vi "Drop Parameters.vi"(6 "Main UI Message Queue":refnum<queue>, 7 "Mouse Position":cluster{"X":i32, "Y":i32}, 8 "error in (no error)":errorcluster, 9 "Parent Window Title":string, 10 "Module Type":T1=enum."Feed", 11 "State in":T2 {"Main Config"."PR Module Configs"."Settings"."PID 2 Parameters"."output range"."output low" format="%.2f"; "Main Config"."PR Module Configs"."Settings"."PID 2 Parameters"."output range"."output high" min=0.0 max=100.0 format="%.2f"; "Main Config"."PR Module Configs"."Settings"."PID 2 Parameters"."PID gains"."derivative time (Td, min)" format="%.3f"; "Main Config"."PR Module Configs"."Settings"."PID 2 Parameters"."PID gains"."integral time (Ti, min)" format="%.3f"; "Main Config"."PR Module Configs"."Settings"."PID 2 Parameters"."PID gains"."proportional gain (Kc)" format="%.3f"; "Main Config"."Steps"."Control" items=["Pump %", "Setpoint"]; "Main Config"."TCU Module Configs"."Settings"."Huber Unistat 410 Settings"."Address" min=0 max=99 format="%02.0f"; "Main Config"."TCU Module Configs"."Settings"."Julabo FP-50 Settings"."Pump Power" min=0 max=8 step=1; "Main Config"."TCU Module Configs"."Settings"."Lauda Settings"."Pump Power" min=0 max=8 step=1; "Main Config"."Flow Module Configs"."Settings"."Bronkhorst M14 Settings"."Smoothing Steps" min=1 step=1; "Main Config"."Flow Module Configs"."Settings"."Bronkhorst M13 Settings"."Smoothing Steps" min=1 step=1; "Main Config"."Pump Module Configs"."Settings"."Ismatech 3 Channel Settings"."Channel Number" min=0 max=3; "Main Config"."Pump Module Configs"."Settings"."Ismatech 3 Channel Settings"."Pump Number" min=1; "Main Config"."Pump Module Configs"."Settings"."ASIA Pump C"."channel" min=0 max=1 step=1; "Main Config"."Pump Module Configs"."Settings"."Masterflex"."Pump Number" min=1.0 max=20.0 step=1.0; "Main Config"."Pump Module Configs"."Settings"."Ismatech"."Pump Number" min=1.0 max=20.0 step=1.0; "Main Config"."Feed Module Configs"."Settings"."Bronkhorst M14 Settings"."Smoothing Steps" min=1 step=1; "Main Config"."Feed Module Configs"."Settings"."Ismatech 3 Channel Settings"."Channel Number" min=0 max=3; "Main Config"."Feed Module Configs"."Settings"."Ismatech 3 Channel Settings"."Pump Number" min=1; "Main Config"."Feed Module Configs"."Settings"."PID range"."PID Low" min=0.0 max=100.0 format="%.2f"; "Main Config"."Feed Module Configs"."Settings"."PID range"."PID High" format="%.2f"; "Main Config"."Feed Module Configs"."Settings"."PID 2 Parameters"."PID gains"."derivative time (Td, min)" format="%.3f"; "Main Config"."Feed Module Configs"."Settings"."PID 2 Parameters"."PID gains"."integral time (Ti, min)" format="%.3f"; "Main Config"."Feed Module Configs"."Settings"."PID 2 Parameters"."PID gains"."proportional gain (Kc)" format="%.3f"; "Main Config"."Feed Module Configs"."Settings"."Bronkhorst M13 Flow Meter"."Smoothing Steps" min=1 step=1; "Main Config"."Feed Module Configs"."Settings"."ASIA Pump C"."channel" min=0 max=1 step=1; "Main Config"."Feed Module Configs"."Settings"."Ismatech"."Pump Number" min=1.0 max=20.0 step=1.0; "Main Config"."Feed Module Configs"."Settings"."Masterflex"."Pump Number" min=1.0 max=20.0 step=1.0}) -> (0 "error out":errorcluster, 2 "Drop Parameters":T79, 3 "State out":T2 {"Main Config"."PR Module Configs"."Settings"."PID 2 Parameters"."output range"."output low" format="%.2f"; "Main Config"."PR Module Configs"."Settings"."PID 2 Parameters"."output range"."output high" min=0.0 max=100.0 format="%.2f"; "Main Config"."PR Module Configs"."Settings"."PID 2 Parameters"."PID gains"."derivative time (Td, min)" format="%.3f"; "Main Config"."PR Module Configs"."Settings"."PID 2 Parameters"."PID gains"."integral time (Ti, min)" format="%.3f"; "Main Config"."PR Module Configs"."Settings"."PID 2 Parameters"."PID gains"."proportional gain (Kc)" format="%.3f"; "Main Config"."Steps"."Control" items=["Pump %", "Setpoint"]; "Main Config"."TCU Module Configs"."Settings"."Huber Unistat 410 Settings"."Address" min=0 max=99 format="%02.0f"; "Main Config"."TCU Module Configs"."Settings"."Julabo FP-50 Settings"."Pump Power" min=0 max=8 step=1; "Main Config"."TCU Module Configs"."Settings"."Lauda Settings"."Pump Power" min=0 max=8 step=1; "Main Config"."Flow Module Configs"."Settings"."Bronkhorst M14 Settings"."Smoothing Steps" min=1 step=1; "Main Config"."Flow Module Configs"."Settings"."Bronkhorst M13 Settings"."Smoothing Steps" min=1 step=1; "Main Config"."Pump Module Configs"."Settings"."Ismatech 3 Channel Settings"."Channel Number" min=0 max=3; "Main Config"."Pump Module Configs"."Settings"."Ismatech 3 Channel Settings"."Pump Number" min=1; "Main Config"."Pump Module Configs"."Settings"."ASIA Pump C"."channel" min=0 max=1 step=1; "Main Config"."Pump Module Configs"."Settings"."Masterflex"."Pump Number" min=1.0 max=20.0 step=1.0; "Main Config"."Pump Module Configs"."Settings"."Ismatech"."Pump Number" min=1.0 max=20.0 step=1.0; "Main Config"."Feed Module Configs"."Settings"."Bronkhorst M14 Settings"."Smoothing Steps" min=1 step=1; "Main Config"."Feed Module Configs"."Settings"."Ismatech 3 Channel Settings"."Channel Number" min=0 max=3; "Main Config"."Feed Module Configs"."Settings"."Ismatech 3 Channel Settings"."Pump Number" min=1; "Main Config"."Feed Module Configs"."Settings"."PID range"."PID Low" min=0.0 max=100.0 format="%.2f"; "Main Config"."Feed Module Configs"."Settings"."PID range"."PID High" format="%.2f"; "Main Config"."Feed Module Configs"."Settings"."PID 2 Parameters"."PID gains"."derivative time (Td, min)" format="%.3f"; "Main Config"."Feed Module Configs"."Settings"."PID 2 Parameters"."PID gains"."integral time (Ti, min)" format="%.3f"; "Main Config"."Feed Module Configs"."Settings"."PID 2 Parameters"."PID gains"."proportional gain (Kc)" format="%.3f"; "Main Config"."Feed Module Configs"."Settings"."Bronkhorst M13 Flow Meter"."Smoothing Steps" min=1 step=1; "Main Config"."Feed Module Configs"."Settings"."ASIA Pump C"."channel" min=0 max=1 step=1; "Main Config"."Feed Module Configs"."Settings"."Ismatech"."Pump Number" min=1.0 max=20.0 step=1.0; "Main Config"."Feed Module Configs"."Settings"."Masterflex"."Pump Number" min=1.0 max=20.0 step=1.0})   [LabVIEW 2018, in "Drag and Drop.lvlib"]
uses:
  Drag and Drop.lvlib
  Drop Parameters Cluster.ctl
  support/Message Queue/Message Cluster.ctl
  <vilib>/Utility/miscctls.llb/LVPoint32TypeDef.ctl
  State Cluster.ctl
  Thumbnail Cluster.ctl
  Object Cluster.ctl
  <vilib>/Utility/miscctls.llb/LVRectTypeDef.ctl
  Object Type Enum.ctl
  <vilib>/Utility/miscctls.llb/LVPositionTypeDef.ctl
  Config Module/Controls/Main Config Cluster.ctl
  OPC/OPC Module Config.ctl
  Scale Module Folder/Measure Instrument/State Enum.ctl
  OPC/OPC Settings.ctl
  OPC/Variable Data Cluster.ctl
  <vilib>/OPCUA/controls/NodeId.ctl
  <vilib>/OPCUA/controls/OPC UA StatusCode.ctl
  <vilib>/OPCUA/controls/Subscription ID.ctl
  <vilib>/OPCUA/controls/OPC UA Client Refnum.ctl
  <vilib>/OPCUA/controls/Subscription Data Change.ctl
  <vilib>/OPCUA/controls/Data Type.ctl
  OPC/OPC Tag Data.ctl
  Feed Module/Controls/Feed Module Config Cluster.ctl
  Feed Module/Controls/Feed Module Settings Cluster.ctl
  Ismatec ISM 831C/Controls/Ismatech ISM831C Settings Cluster.ctl
  Masterflex 7550-30/Controls/Settings Cluster.ctl
  Mettler Toledo/Controls/Settings Cluster.ctl
  Bronkhorst M13 Flow Meter/Settings Cluster.ctl
  Measure Instrument/PID 2 Parameters Cluster.ctl
  Measure Instrument/PID Input Enum.ctl
  Measure Instrument/PID 2 Output Enum.ctl
  Tacmina QI/Tacmina QI DAQ Setting.ctl
  KNF Pump/Settings Cluster plus SIMDOS.ctl
  ASIA Pump/Pump Settings.ctl
  VICI M50 Party Mode/Settings Cluster.ctl
  FLOM Pump/Settings Cluster.ctl
  SSI PR Class/SSI PR or LD Settings Cluster.ctl
  Masterflex 75211/Masterflex 75211 DAQ Setting.ctl
  SSI PR Class/SSI P40 Settings Cluster.ctl
  Ismatec 78001/Ismatec 4083.ctl
  Bronkhorst M14 Flow Meter/Settings Cluster.ctl
  Tag VIs/Numeric Alarm Settings Cluster.ctl
  TT Module/Controls/TT Module Config Cluster.ctl
  Acquisition/Hardware Configuration.ctl
  Acquisition/Task Cluster.ctl
  PT Module/Controls/PT Module Config Cluster.ctl
  Scale Module Folder/Feed Module/Controls/Scale Module Config Cluster.ctl
  Scale Module Folder/Feed Module/Controls/Scale Module Settings Cluster.ctl
  Pump Module Folder/Pump Module Config Cluster.ctl
  Pump Module Folder/Pump Module Settings Cluster.ctl
  LabJack Module/Controls/U3 Module Config Cluster.ctl
  Decoration Module/Decoration Module Config Cluster.ctl
  Flow Module Folder/Feed Module/Controls/Flow Module Config Cluster.ctl
  Flow Module Folder/Feed Module/Controls/Flow Module Settings Cluster.ctl
  TCU Module/TCU Module Folder/TCU Module Config Cluster.ctl
  TCU Module/TCU Module Folder/TCU Module Settings Cluster.ctl
  TCU Module/TCU Module Folder/Measure Instrument/Output Devices.ctl
  Huber TCU/Huber Settings.ctl
  Lauda Integral XT-150 TCU/Lauda Settings.ctl
  Julabo Type 1 TCU/Julabo Type 1 TCU Folder/Julabo FP-50 Settings.ctl
  Huber Unistat 410 TCU/Huber Unistat 410 RS485 Settings.ctl
  D-O Module Folder/Not Sure Where this is Used.ctl
  Sequencing/Squence Control.ctl
  D-O Module Folder/D-O Module Config Cluster.ctl
  D-O Module Folder/Valve Clusters.ctl
  D-O Module Folder/D-O Module Settings Cluster.ctl
  D-O Module Folder/D-O Device Settings Cluster.ctl
  VICI Electronic Actuator/VICI Electronic Actuator Settings.ctl
  Pressure Regulator Control Module/Pressure Regulator/Controls/4-20mA Module Config Cluster.ctl
  Pressure Regulator Control Module/Pressure Regulator/Controls/4-20mA Module Settings Cluster.ctl
  Pressure Transmitter/Pressure Transmitter Device Settings.ctl
  Pressure Reg Module/Pressure Regulator Device Settings.ctl
  Sonicator Module Folder/Feed Module/Controls/Sonicator Module Config Cluster.ctl
  Sonicator Module Folder/Feed Module/Controls/Sonicator Module Settings Cluster.ctl
  Sonic Systems P100/Sonic Systems P100 Settings.ctl
  Agitator Module Folder/Feed Module/Controls/Agitator Module Config Cluster.ctl
  Agitator Module Folder/Feed Module/Controls/Agitator Module Settings Cluster.ctl
  IKA EUROSTAR/IKA EUROSTAR Settings.ctl
  Centrifuge Module Folder/Centrifuge Module Config Cluster.ctl
  Centrifuge Module Folder/Centrifuge Module Settings Cluster.ctl
  EPOS4/Controls/Device Selection.ctl
  EPOS4/Controls/EPOS Communication Settings.ctl
  Module Type Enum.ctl
  Module Instance Number Operation Enum.ctl
  Flow Module Folder/Flow Module (Main).vi
  D-O Module Folder/D-O Module (Main).vi
  TCU Module/TCU Module Folder/TCU Module (Main).vi
  LabJack Module/U3 (Main).vit
  Sonicator Module Folder/Sonicator Module (Main).vi
  Agitator Module Folder/Agitator Module (Main).vi
  Centrifuge Module Folder/Centrifuge Module (Main).vi
  Feed Module/Feed Module.lvlib
  TT Module/TT Module.lvlib
  support/Message Queue/Message Queue.lvlib
  Bronkhorst M13 Flow Meter/Bronkhorst M13 Flow Meter.lvlib
  Mettler Toledo/Mettler Toledo.lvlib
  Masterflex 7550-30/Masterflex 7550-30.lvlib
  Ismatec ISM 831C/Ismatec ISM 831C.lvlib
  PT Module/PT Module.lvlib
  Shared Variables/Dynamic Shared Variables.lvlib
  Scale Module Folder/Scale Module.lvlib
  Pump Module Folder/Pump Module.lvlib
  LabJack Module/U3 Module.lvlib
  Flow Module Folder/Flow Module.lvlib
  Tacmina QI/Tacmina QI.lvlib
  KNF Pump/KNF SIMDOS.lvlib
  TCU Module/TCU Module Folder/TCU Module.lvlib
  Huber TCU/Huber Ministat 230 TCU.lvlib
  Lauda Integral XT-150 TCU/Lauda TCU.lvlib
  Julabo Type 1 TCU/Julabo Type 1 TCU Folder/Julabo Type FP-50 TCU.lvlib
  ASIA Pump.lvlib
  VICI M50 Party Mode/VICI M6 M50 Party Mode.lvlib
  D-O Module Folder/D-O Module.lvlib
  Pressure Regulator Control Module/Pressure Regulator/4-20mA Module.lvlib
  Pressure Transmitter/Pressure Transmitter Library.lvlib
  Pressure Reg Module/Pressure Regulator Library.lvlib
  FLOM Pump/FLOM Pump.lvlib
  SSI PR Class/SSI PR or LD Pump.lvlib
  OPC/OPC UA.lvlib
  Scale Module Folder/Measure Instrument/Scale Module Engine.lvlib
  D-O Module Folder/DIO Valve/VICI Electronic Actuator.lvlib
  Masterflex 75211/Masterflex 75211.lvlib
  SSI PR Class/SSI P40 Pump.lvlib
  Huber Unistat 410 TCU/Huber Unistat 410 TCU.lvlib
  Ismatec 78001/Ismatec 4308.lvlib
  Bronkhorst M14 Flow Meter/Bronkhorst M14 Flow Meter.lvlib
  Sonicator Module Folder/Sonicator Module.lvlib
  Sonic Systems P100/Sonic Systems P100.lvlib
  Agitator Module Folder/Agitator Module.lvlib
  Centrifuge Module Folder/Centrifuge Module.lvlib
  EPOS4/EPOS4.lvlib
  IKA EUROSTAR/IKA EUROSTAR.lvlib
  Config Module/Config Module.lvlib
  DAQ/DAQ.lvlib
  Sequencing/Sequencing Library.lvlib
panel:
  # "Agitator Settings"
  # "Sonicator Settings"
  # "Instrument Settings"
  # "Instrument Settings"
  # "Output Instruments"
  # "Flow Meter Settings"
  # "Output Instruments"
  # "Scale Settings"
  # "Output Instruments"
  # "Input Instruments"
  # "Agitator Settings"
  # "Sonicator Settings"
  # "Instrument Settings"
  # "Instrument Settings"
  # "Output Instruments"
  # "Flow Meter Settings"
  # "Output Instruments"
  # "Scale Settings"
  # "Output Instruments"
  # "Input Instruments"
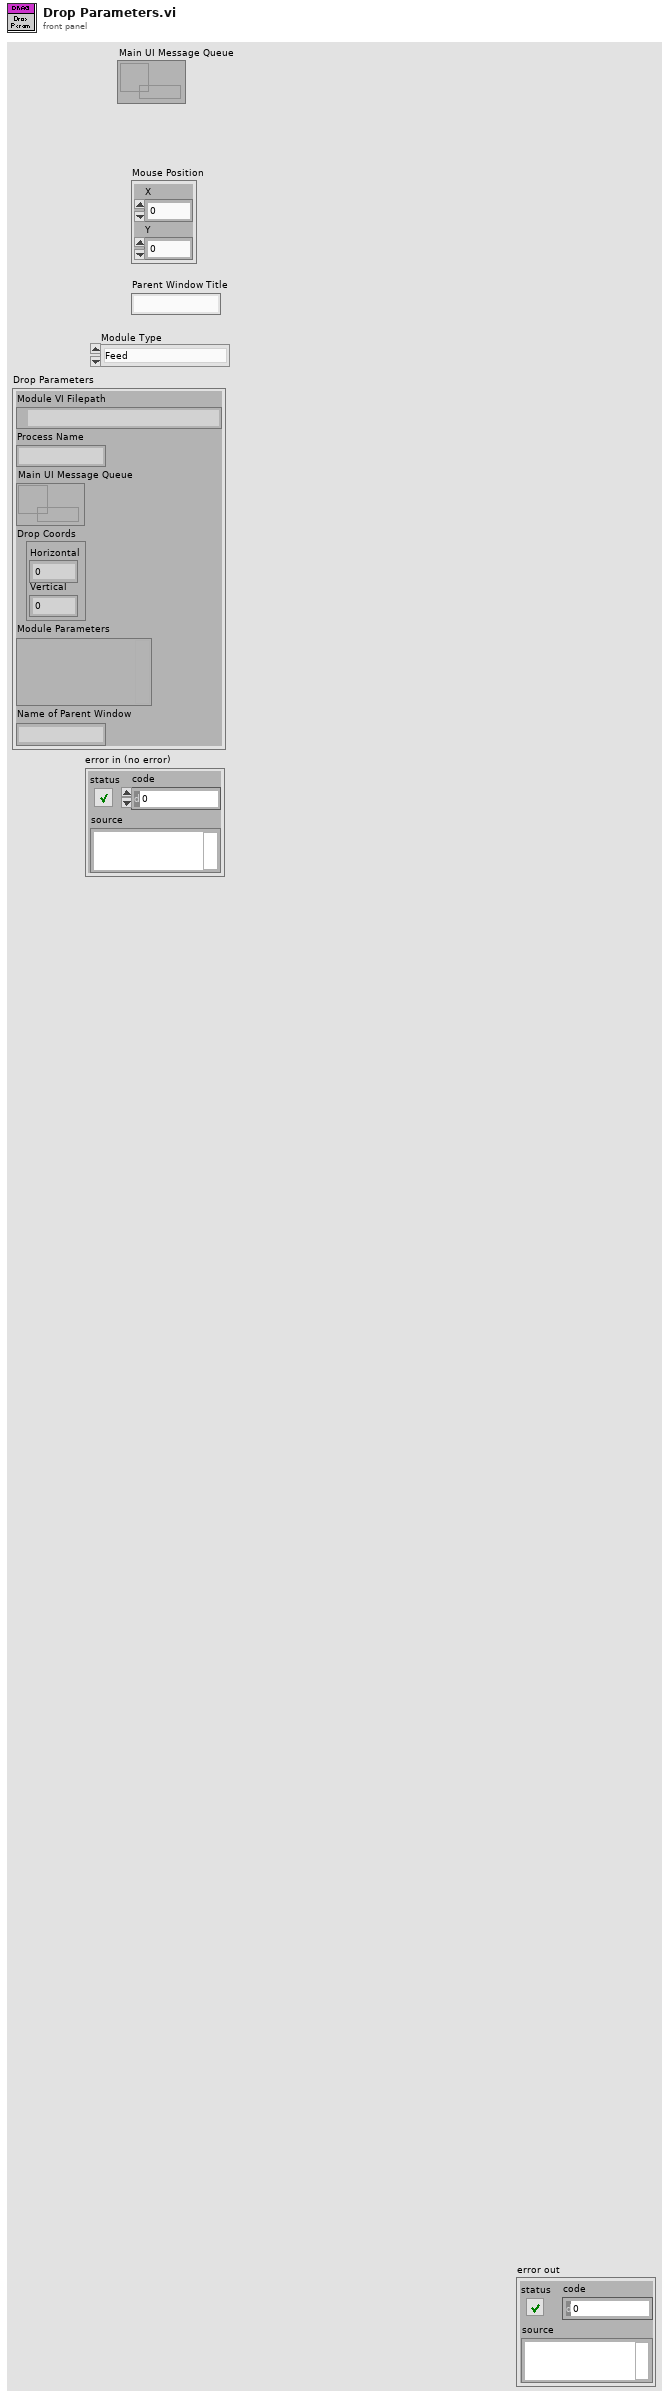
[diagram p1: front panel]
types:
  T1 = typedef "Drag and Drop.lvlib/Module Type Enum.ctl" = enum16{"<unknown module>", "Feed", "TT", "PT", "Scale", "Flow", "Pump", "U3", "TCU", "DO", "PR", "OPC", "SC", "AM", "CM"}
  T2 = typedef "Drag and Drop.lvlib/State Cluster.ctl" = cluster{"VI refs":refnum<vi>[], "Queues":refnum<queue>[], "[Thumbnails]":T3[], "Drag Object Idx":i32, "[Objects]":T4[], "Active Object":i32, "Drop Offset":T7, "Process Name":string, "Main Config":T8, "Campaign Filepath":path, "Config Changed?":bool}
  T3 = typedef "Thumbnail Cluster.ctl" = cluster{"Path":path, "Rectangle":cluster{"left":i16, "top":i16, "right":i16, "bottom":i16}}
  T4 = typedef "Object Cluster.ctl" = cluster{"BMP Path":path, "Anchor Position":cluster{"X":i32, "Y":i32}, "Hot Spot":T5, "Type":T6, "Parameters":variant}
  T5 = typedef "LVRectTypeDef.ctl" = cluster{"Left":i16, "Top":i16, "Right":i16, "Bottom":i16}
  T6 = typedef "Object Type Enum.ctl" = enum16{"Icon", "Line", "Text", "Feed Module"}
  T7 = typedef "LVPositionTypeDef.ctl" = cluster{"Left":i32, "Top":i32}
  T8 = typedef "Config Module.lvlib/Main Config Cluster.ctl" = cluster{"Notebook":string, "OPC Module Configs":T9[], "Feed Module Configs":T19[], "Log File Path":path, "TT Module Configs":T39[], "DAQ Config":T40, "PT Module Configs":T42[], "Scale Module Configs":T43[], "Pump Module Configs":T45[], "U3 Module Configs":T47[], "Decoration Module Configs":T48[], "Flow Module Configs":T49[], "TCU Module Configs":T51[], "Steps":T58, "Abort":bool, "DO Module Configs":T60[], "PR Module Configs":T65[], "SC Module Configs":T69[], "AM Module Configs":T72[], "CM Module Configs":T75[], "Cycle Period":dbl}
  T9 = typedef "OPC UA.lvlib/OPC Module Config.ctl" = cluster{"State":T10, "GUID":string, "Process Name":string, "User name":string, "Drop Coords":T11, "Configuration":T12, "First Iteration":bool, "Data":cluster{"Object Name":string, "Variable Array":T13[]}[], "Load Count":i32, "Log Started":bool, "subscription ID out":T16, "OPC UA client refnum out":T17, "Event Registration Refnum":refnum<event-registration>, "Start Time":timestamp, "Current Time":timestamp, "Tag Data":T18[]}
  T10 = typedef "Scale Module.lvlib/Scale Module Engine.lvlib/State Enum.ctl" = enum16{"Measuring", "Idle"}
  T11 = typedef "LVPoint32TypeDef.ctl" = cluster{"Horizontal":i32, "Vertical":i32}
  T12 = typedef "OPC UA.lvlib/OPC Settings.ctl" = cluster{"Cycle Period":dbl, "server endpoint URL":string, "security policy":cluster{"message mode":enum16{"None", "Sign", "Sign and Encrypt"}, "security":enum16{"Basic256", "Basic128Rsa15"}}, "Trust Any Server":bool}
  T13 = typedef "OPC UA.lvlib/Variable Data Cluster.ctl" = cluster{"node ID":T14, "browse name":string, "status":T15, "timestamp":timestamp, "value ":variant}
  T14 = typedef "NodeId.ctl" = string
  T15 = typedef "OPC UA StatusCode.ctl" = u32
  T16 = typedef "Subscription ID.ctl" = u32
  T17 = typedef "OPC UA Client Refnum.ctl" = refnum<k21>
  T18 = typedef "OPC UA.lvlib/OPC Tag Data.ctl" = cluster{"Include this Device":bool, "Device Name":string, "OPC Tag Data":cluster{"Tag":string, "Value":variant, "Time Stamp":timestamp}[]}
  T19 = typedef "Feed Module.lvlib/Feed Module Config Cluster.ctl" = cluster{"GUID":string, "Drop Coords":T11, "Process Name":string, "User name":string, "Queue Name":string, "Settings":T20, "Settings Load Count":i32, "OP Load Count":i32}
  T20 = typedef "Feed Module.lvlib/Feed Module Settings Cluster.ctl" = cluster{"Cycle Period":dbl, "Ismatech":T21, "Masterflex":T22, "Mettler":T23, "Bronkhorst M13 Flow Meter":T24, "PID 2 Parameters":T25, "Manual Entry":dbl, "Auto?":bool, "PID range":cluster{"PID High":dbl, "PID Low":dbl, "High Warning":dbl}, "Tacmina Settings":T28, "KNF SIMDOS Settings":T29, "ASIA Pump C":T30, "VICI Settings":T31, "FLOM Settings":T32, "SSI PR/LD Settings":T33, "Masterflex 75211 Settings":T34, "SSI P40 Settings":T35, "Ismatech 3 Channel Settings":T36, "Bronkhorst M14 Settings":T37, "Reset Totalizer":bool, "Input Num Alarm Settings":T38[], "Control Type":enum32{"g/min", "ml/min"}, "Front End Display Options":cluster{"Temperature":bool, "Scale Grams":bool, "Density":bool, "Flow (g/min)":bool, "Flow (ml/min)":bool, "PSIG":bool, "Total Grams":bool, "Updated":bool}}
  T21 = typedef "Ismatec ISM 831C.lvlib/Ismatech ISM831C Settings Cluster.ctl" = cluster{"VISA resource name":refnum<visa-resource-name>, "Simulated?":bool, "Pump Number":dbl, "Reverse?":bool}
  T22 = typedef "Masterflex 7550-30.lvlib/Settings Cluster.ctl" = cluster{"VISA resource name":refnum<visa-resource-name>, "Simulated?":bool, "Pump Number":dbl, "Reverse?":bool}
  T23 = typedef "Mettler Toledo.lvlib/Settings Cluster.ctl" = cluster{"VISA resource name":refnum<visa-resource-name>, "Simulated?":bool}
  T24 = typedef "Bronkhorst M13 Flow Meter.lvlib/Settings Cluster.ctl" = cluster{"VISA resource name":refnum<visa-resource-name>, "Simulated?":bool, "Smoothing Steps":i32}
  T25 = typedef "PID 2 Parameters Cluster.ctl" = cluster{"Input Device":T26, "Output Device":T27, "Setpoint":dbl, "PID gains":cluster{"proportional gain (Kc)":dbl, "integral time (Ti, min)":dbl, "derivative time (Td, min)":dbl}}
  T26 = typedef "PID Input Enum.ctl" = enum16{"Default", "Bronkhorst M13", "Bronkhorst M14", "Scale Rate of Change"}
  T27 = typedef "PID 2 Output Enum.ctl" = enum16{"Default", "Ismatec ISM 4308", "Ismatec ISM 831C", "Masterflex 7550-30", "VICI M6", "VICI M50", "Tacmina QI", "KNF SIMDOS", "ASIA Type C", "FLOM UI-22-11", "SSI PR/LD", "SSI P40", "Masterflex 75211-70"}
  T28 = typedef "Tacmina QI.lvlib/Tacmina QI DAQ Setting.ctl" = cluster{"Analog DAQ Task":refnum<k21>, "Digital DAQ Task":refnum<k21>}
  T29 = typedef "KNF SIMDOS.lvlib/Settings Cluster plus SIMDOS.ctl" = cluster{"VISA resource name":refnum<visa-resource-name>, "Simulated?":bool}
  T30 = typedef "ASIA Pump.lvlib/Pump Settings.ctl" = cluster{"ASIA Pump #":i32, "channel":i32, "Simulated":bool}
  T31 = typedef "VICI M6 M50 Party Mode.lvlib/Settings Cluster.ctl" = cluster{"VISA resource name":refnum<visa-resource-name>, "Pump ID":string, "Pump Head Vol":dbl, "Reverse?":bool, "Simulated?":bool}
  T32 = typedef "FLOM Pump.lvlib/Settings Cluster.ctl" = cluster{"VISA resource name":refnum<visa-resource-name>, "Simulated?":bool, "Pump Number":dbl}
  T33 = typedef "SSI PR or LD Pump.lvlib/SSI PR or LD Settings Cluster.ctl" = cluster{"VISA resource name":refnum<visa-resource-name>, "Simulated?":bool}
  T34 = typedef "Masterflex 75211.lvlib/Masterflex 75211 DAQ Setting.ctl" = cluster{"Analog DAQ Task":refnum<k21>, "Digital DAQ Task":refnum<k21>}
  T35 = typedef "SSI P40 Pump.lvlib/SSI P40 Settings Cluster.ctl" = cluster{"VISA resource name":refnum<visa-resource-name>, "Simulated?":bool}
  T36 = typedef "Ismatec 4308.lvlib/Ismatec 4083.ctl" = cluster{"VISA resource name":refnum<visa-resource-name>, "Pump Number":i16, "Channel Number":i16, "Simulated?":bool, "Reverse?":bool}
  T37 = typedef "Bronkhorst M14 Flow Meter.lvlib/Settings Cluster.ctl" = cluster{"VISA resource name":refnum<visa-resource-name>, "Simulated?":bool, "Smoothing Steps":i32}
  T38 = typedef "Numeric Alarm Settings Cluster.ctl" = cluster{"enable? (F)":bool, "name":string, "alarm type":enum16{"HI_HI", "HI", "LO", "LO_LO"}, "level/change":dbl, "deadband/time":dbl, "alarm delay":dbl, "priority":u32, "ack type":enum16{"Auto", "User", "None", "Each Occurrence"}, "area":string, "description":string, "log? (T)":bool}
  T39 = typedef "TT Module.lvlib/TT Module Config Cluster.ctl" = cluster{"GUID":string, "Drop Coords":T11, "Input Channel Tag Name ":string, "Process Name":string, "User name":string, "Queue Name":string, "Input Channel Numeric Alarm Settings":T38[]}
  T40 = typedef "DAQ.lvlib/Hardware Configuration.ctl" = cluster{"Tasks Array":T41[]}
  T41 = typedef "Task Cluster.ctl" = cluster{"DAQmx Task":refnum<k21>, "Read-Write Radio":enum32{"Read", "Write"}}
  T42 = typedef "PT Module.lvlib/PT Module Config Cluster.ctl" = cluster{"GUID":string, "Drop Coords":T11, "Input Channel Tag Name ":string, "Process Name":string, "User name":string, "Queue Name":string, "Input Channel Numeric Alarm Settings":T38[]}
  T43 = typedef "Scale Module.lvlib/Scale Module Config Cluster.ctl" = cluster{"GUID":string, "Drop Coords":T11, "Process Name":string, "User name":string, "Queue Name":string, "Settings":T44, "Load Count":i32}
  T44 = typedef "Scale Module.lvlib/Scale Module Settings Cluster.ctl" = cluster{"Cycle Period":dbl, "Mettler":T23, "Scale Type":string}
  T45 = typedef "Pump Module.lvlib/Pump Module Config Cluster.ctl" = cluster{"GUID":string, "Drop Coords":T11, "Process Name":string, "User name":string, "Queue Name":string, "Settings":T46, "Load Count":i32}
  T46 = typedef "Pump Module.lvlib/Pump Module Settings Cluster.ctl" = cluster{"Cycle Period":dbl, "Manual Entry":dbl, "Output Device":T27, "Ismatech":T21, "Ismatech 3 Channel Settings":T36, "Masterflex":T22, "VICI Settings":T31, "Tacmina Settings":T28, "KNF SIMDOS Settings":T29, "ASIA Pump C":T30, "FLOM Settings":T32, "SSI PR/LD Settings":T33, "SSI P40 Settings":T33, "Masterflex 75211 Settings":T34, "Pump Calibration File":path, "Calibration Slope":dbl, "Calibration Y Intercept":dbl, "Pump Cal Enum":u16, "Reset Totalizer":bool}
  T47 = typedef "U3 Module.lvlib/U3 Module Config Cluster.ctl" = cluster{"GUID":string, "Drop Coords":T11, "AI Channel Number":enum16{"Default", "AI0", "AI1", "AI2", "AI3", "AI4", "AI5", "AI6", "AI7"}, "Process Name":string, "User name":string, "Queue Name":string, "Input Channel Numeric Alarm Settings":T38[]}
  T48 = typedef "Decoration Module Config Cluster.ctl" = cluster{"GUID":string, "Drop Coords":T11, "Decoration Filepath":path}
  T49 = typedef "Flow Module.lvlib/Flow Module Config Cluster.ctl" = cluster{"GUID":string, "Drop Coords":T11, "Process Name":string, "User name":string, "Queue Name":string, "Settings":T50, "Load Count":i32}
  T50 = typedef "Flow Module.lvlib/Flow Module Settings Cluster.ctl" = cluster{"Cycle Period":dbl, "Flow Meter Type":string, "Bronkhorst M13 Settings":T24, "Bronkhorst M14 Settings":T37, "Reset Totalizer":bool}
  T51 = typedef "TCU Module.lvlib/TCU Module Config Cluster.ctl" = cluster{"GUID":string, "Drop Coords":T11, "Process Name":string, "User name":string, "Queue Name":string, "Settings":T52, "Load Count":i32, "Power Level Changed":bool}
  T52 = typedef "TCU Module.lvlib/TCU Module Settings Cluster.ctl" = cluster{"Cycle Period":dbl, "Setpoint Entry":dbl, "Output Device":T53, "Huber Ministat 230 Settings":T54, "Lauda Settings":T55, "Julabo FP-50 Settings":T56, "Internal Control?":bool, "Huber Unistat 410 Settings":T57}
  T53 = typedef "Output Devices.ctl" = enum16{"Default", "Huber Ministat 230", "Huber Unistat 410", "Lauda XT-150", "Julabo FP-50"}
  T54 = typedef "Huber Ministat 230 TCU.lvlib/Huber Settings.ctl" = cluster{"VISA resource name":refnum<visa-resource-name>, "Simulated?":bool}
  T55 = typedef "Lauda TCU.lvlib/Lauda Settings.ctl" = cluster{"VISA resource name":refnum<visa-resource-name>, "Simulated?":bool, "Pump Power":i32}
  T56 = typedef "Julabo Type FP-50 TCU.lvlib/Julabo FP-50 Settings.ctl" = cluster{"VISA resource name":refnum<visa-resource-name>, "Simulated?":bool, "Pump Power":i32}
  T57 = typedef "Huber Unistat 410 TCU.lvlib/Huber Unistat 410 RS485 Settings.ctl" = cluster{"VISA resource name":refnum<visa-resource-name>, "Address":i8, "Simulated?":bool}
  T58 = typedef "Not Sure Where this is Used.ctl" = T59[]
  T59 = typedef "Sequencing Library.lvlib/Squence Control.ctl" = cluster{"Module":string, "Control":u16, "Value":dbl, "Wait (sec)":dbl}
  T60 = typedef "D-O Module.lvlib/D-O Module Config Cluster.ctl" = cluster{"GUID":string, "Drop Coords":T11, "Process Name":string, "User name":string, "Queue Name":string, "Settings":T61, "Load Count":i32}
  T61 = typedef "D-O Module.lvlib/Valve Clusters.ctl" = cluster{"Valve Settings":T62, "Valve Type":enum16{"Default", "Digital Output Valve", "VICI Electronic Actuator"}, "Time On (Sec)":dbl, "Time Off (Sec)":dbl, "Run?":bool}
  T62 = typedef "D-O Module.lvlib/D-O Module Settings Cluster.ctl" = cluster{"D-O Settings":T63, "VICI Electronic Actuator":T64}
  T63 = typedef "D-O Module.lvlib/D-O Device Settings Cluster.ctl" = cluster{"DAQmx Task Name":refnum<k21>, "Output Channel":u16, "Output Channel Names":string[]}
  T64 = typedef "VICI Electronic Actuator.lvlib/VICI Electronic Actuator Settings.ctl" = cluster{"VISA resource name":refnum<visa-resource-name>, "Mode":enum16{"Two Positions With Stops", "Two Positions Without Stops", "Mutiposition"}, "Simulated":bool}
  T65 = typedef "4-20mA Module.lvlib/4-20mA Module Config Cluster.ctl" = cluster{"GUID":string, "Drop Coords":T11, "Process Name":string, "User name":string, "Queue Name":string, "Settings":T66, "Settings Load Count":i32}
  T66 = typedef "4-20mA Module.lvlib/4-20mA Module Settings Cluster.ctl" = cluster{"Cycle Period":dbl, "PID 2 Parameters":cluster{"Input Device":enum16{"Default", "4-20mA"}, "Output Device":enum16{"Default", "Equilibar Pressure Reg", "Flow Regulator"}, "Setpoint":dbl, "PID gains":cluster{"proportional gain (Kc)":dbl, "integral time (Ti, min)":dbl, "derivative time (Td, min)":dbl}, "output range":cluster{"output low":dbl, "output high":dbl}}, "Manual Entry":dbl, "Auto?":bool, "4-20mA Input Settings":T67, "4-20mA Out Settings":T68, "Input Channel Tag Name ":string}
  T67 = typedef "Pressure Transmitter Library.lvlib/Pressure Transmitter Device Settings.ctl" = cluster{"Input Channel ":u16}
  T68 = typedef "Pressure Regulator Library.lvlib/Pressure Regulator Device Settings.ctl" = cluster{"Output DAQ Task":refnum<k21>}
  T69 = typedef "Sonicator Module.lvlib/Sonicator Module Config Cluster.ctl" = cluster{"GUID":string, "Drop Coords":T11, "Process Name":string, "User name":string, "Queue Name":string, "Settings":T70, "Load Count":i32}
  T70 = typedef "Sonicator Module.lvlib/Sonicator Module Settings Cluster.ctl" = cluster{"Cycle Period":dbl, "Sonicator Type":string, "SS P100 Settings":T71, "Setpoint (µm)":dbl, "Cutoff (W)":dbl}
  T71 = typedef "Sonic Systems P100.lvlib/Sonic Systems P100 Settings.ctl" = cluster{"VISA resource name":refnum<visa-resource-name>, "Simulated?":bool}
  T72 = typedef "Agitator Module.lvlib/Agitator Module Config Cluster.ctl" = cluster{"GUID":string, "Drop Coords":T11, "Process Name":string, "User name":string, "Queue Name":string, "Settings":T73, "Load Count":i32}
  T73 = typedef "Agitator Module.lvlib/Agitator Module Settings Cluster.ctl" = cluster{"Cycle Period":dbl, "Agitator Type":string, "Setpoint (µm)":dbl, "IKA EUROSTAR Settings":T74}
  T74 = typedef "IKA EUROSTAR.lvlib/IKA EUROSTAR Settings.ctl" = cluster{"VISA resource name":refnum<visa-resource-name>, "Simulated?":bool}
  T75 = typedef "Centrifuge Module.lvlib/Centrifuge Module Config Cluster.ctl" = cluster{"GUID":string, "Drop Coords":T11, "Process Name":string, "User name":string, "Queue Name":string, "Settings":T76, "Load Count":i32}
  T76 = typedef "Centrifuge Module.lvlib/Centrifuge Module Settings Cluster.ctl" = cluster{"Cycle Period":dbl, "Manual Entry":dbl, "Output Device":T77, "EPOS4 Settings":T78}
  T77 = typedef "Device Selection.ctl" = enum16{"Default", "EPOS4"}
  T78 = typedef "EPOS4.lvlib/EPOS Communication Settings.ctl" = cluster{"VISA resource name":refnum<visa-resource-name>, "axis":cluster{"keyHandle":u32, "nodeId":u16}, "Simulated?":bool}
  T79 = typedef "Drop Parameters Cluster.ctl" = cluster{"Module VI Filepath":path, "Process Name":string, "Main UI Message Queue":refnum<queue>, "Drop Coords":T11, "Module Parameters":variant, "Name of Parent Window":string}
  T80 = typedef "Module Instance Number Operation Enum.ctl" = enum16{"Init", "Next Instance Number"}
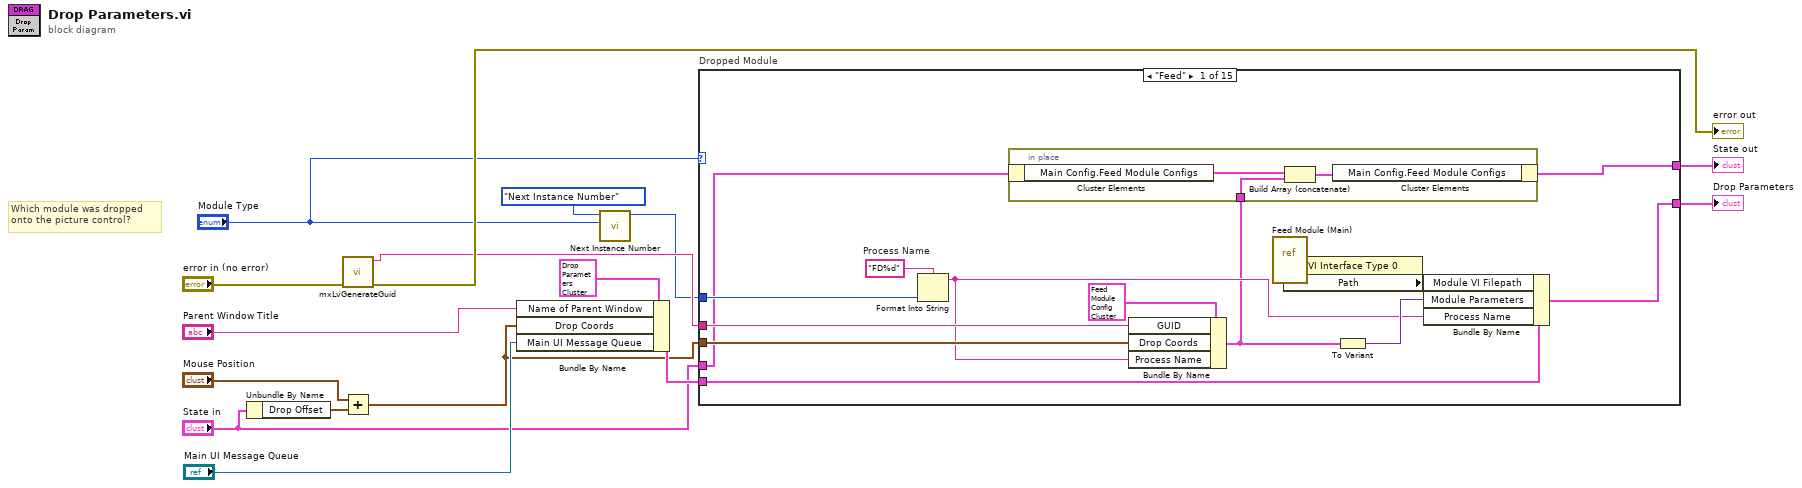
[diagram p0: block diagram]
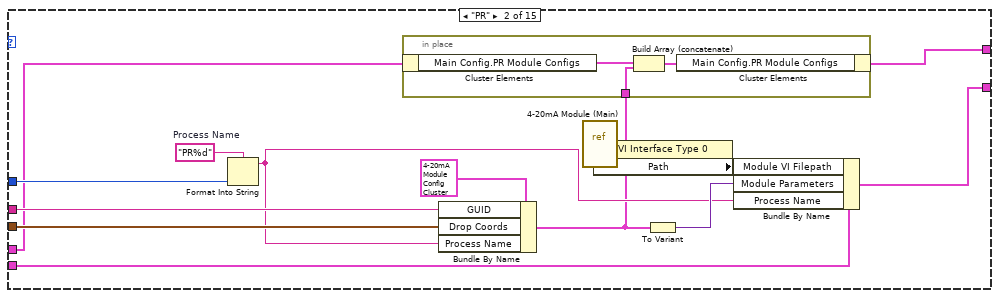
[diagram p2: hidden frame]
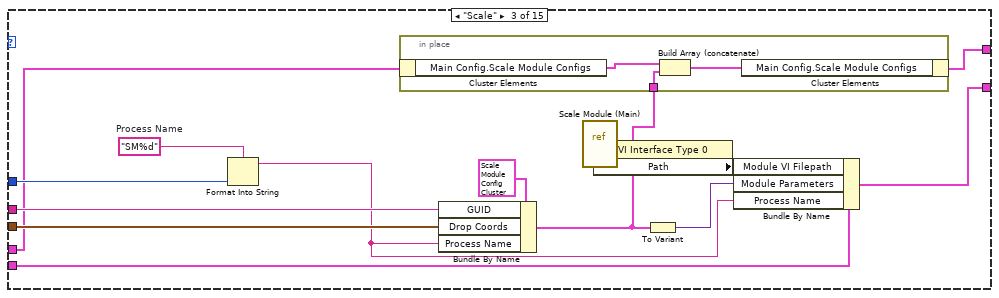
[diagram p3: hidden frame]
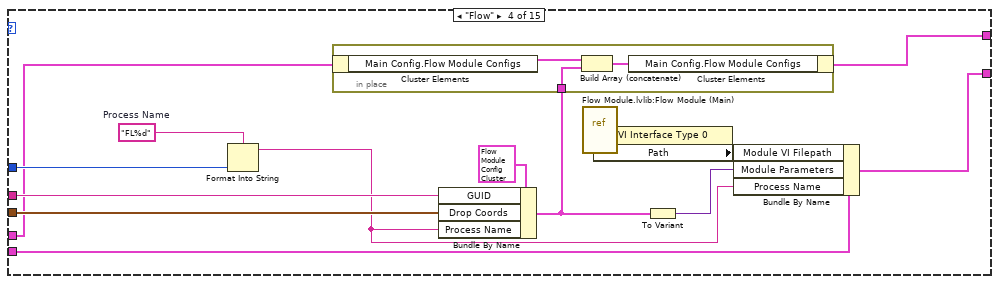
[diagram p4: hidden frame]
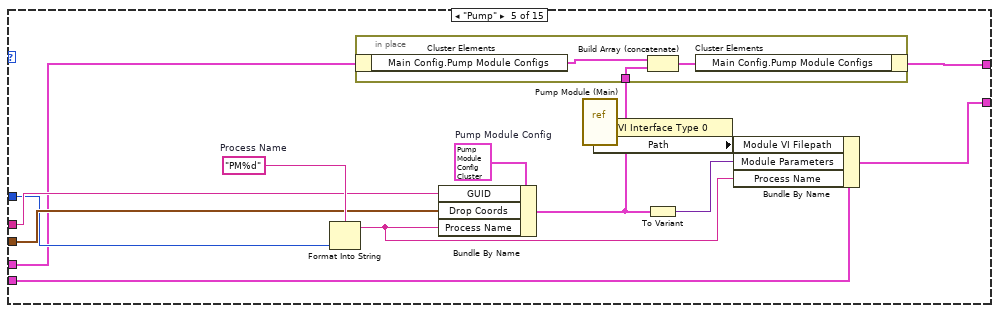
[diagram p5: hidden frame]
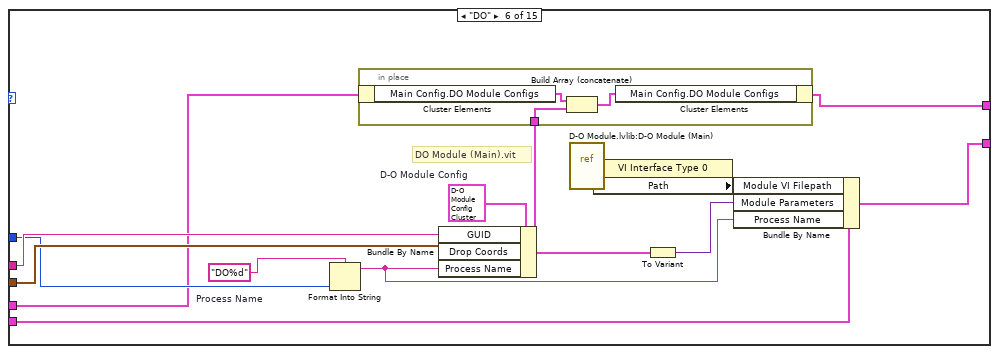
[diagram p6: hidden frame]
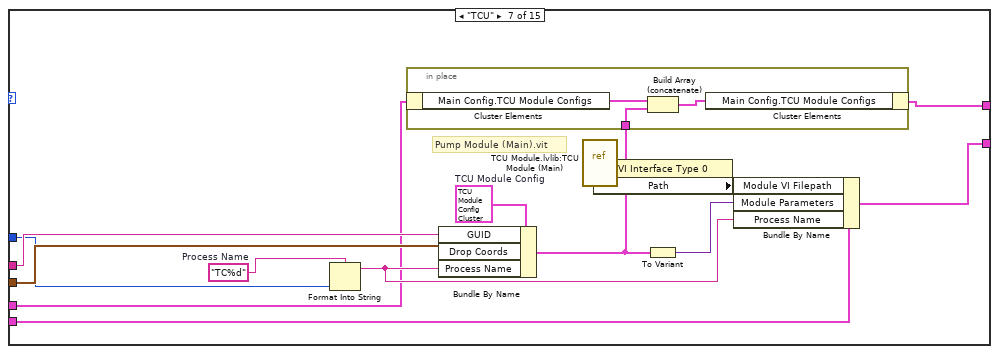
[diagram p7: hidden frame]
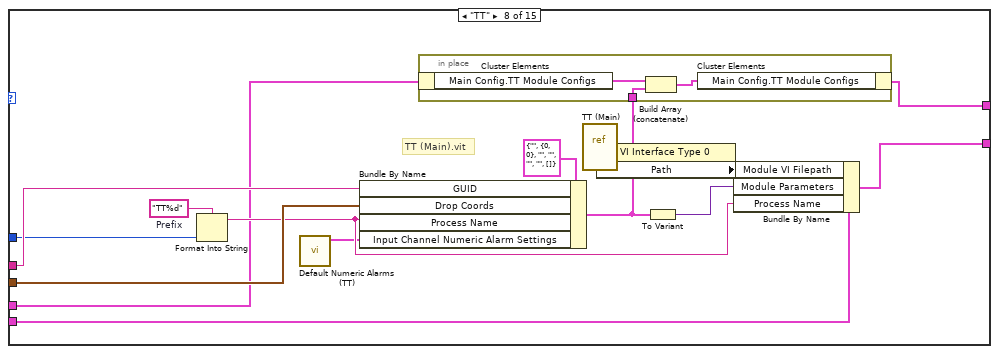
[diagram p8: hidden frame]
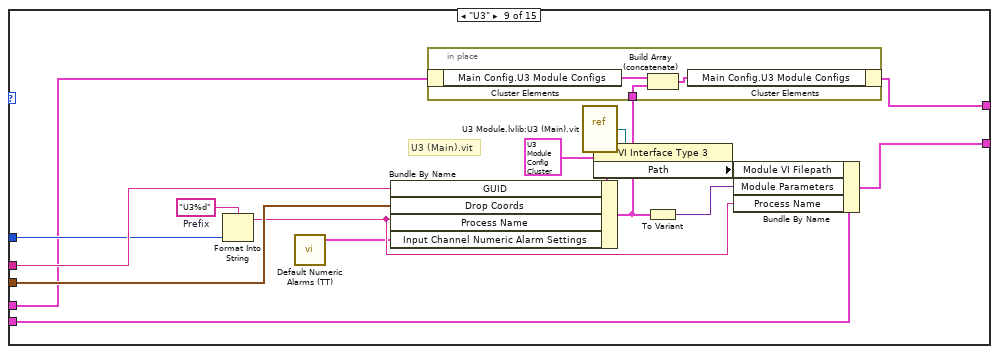
[diagram p9: hidden frame]
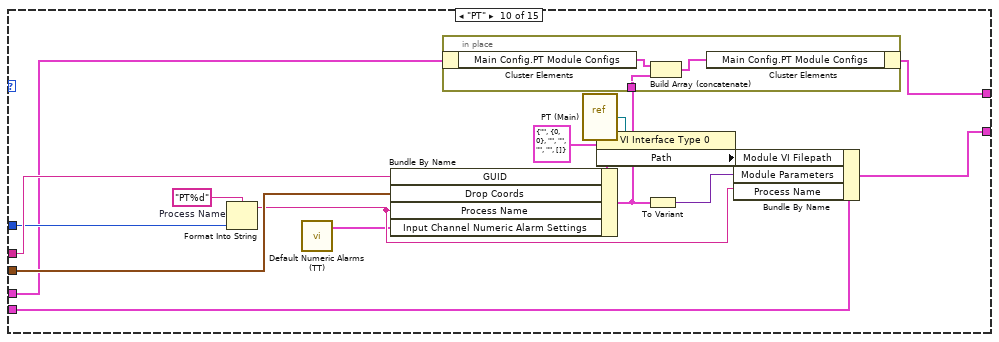
[diagram p10: hidden frame]
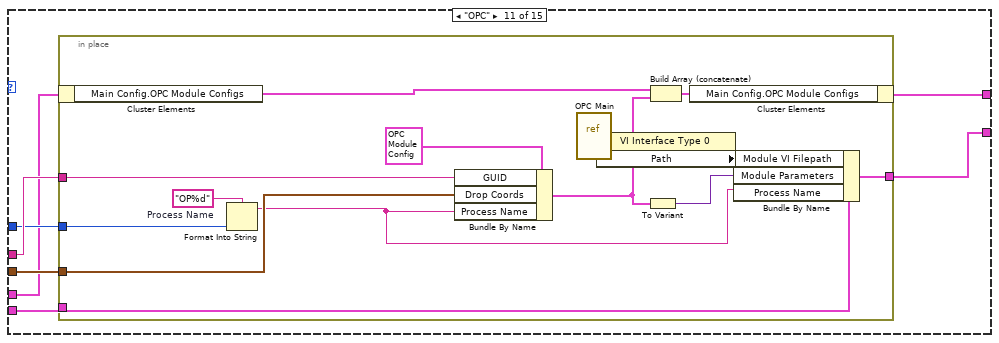
[diagram p11: hidden frame]
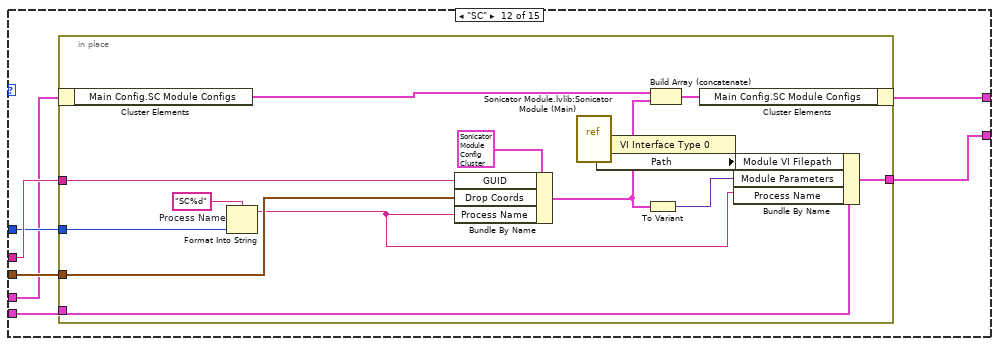
[diagram p12: hidden frame]
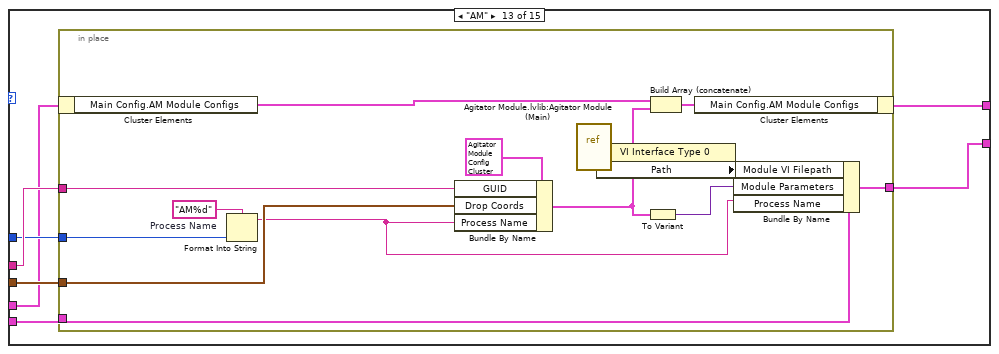
[diagram p13: hidden frame]
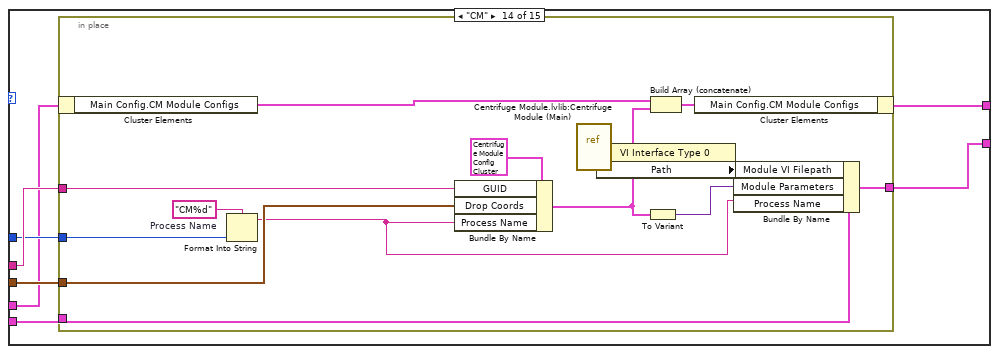
[diagram p14: hidden frame]
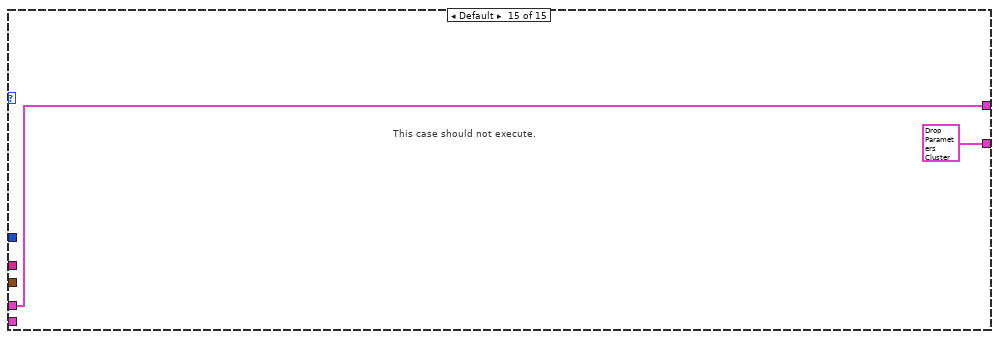
[diagram p15: hidden frame]
diagram:
  # "Which module was dropped\nonto the picture control?"
  n1 = Unbundle By Name("State in") -> ("Drop Offset"=w12:T7)
  n2 = call <resource>:"mxLvGenerateGuid.vi"("Error In"="error in (no error)") -> ("Error Out"=→"error out":errorcluster, "Value"=w13:string)  [unwired: 9 in]
  n3 = Add(x="Mouse Position", y=w12) -> (x+y=w6:T7)
  n4 = Bundle By Name(cluster=T79 {"Module VI Filepath"=path "", "Process Name"="", "Main UI Message Queue"=refnum, "Drop Coords"={"Horizontal"=0, "Vertical"=0}, "Module Parameters"=variant, "Name of Parent Window"=""} ("Drop Parameters"), "Name of Parent Window"="Parent Window Title", "Drop Coords"=w6, "Main UI Message Queue"="Main UI Message Queue") -> (w8:T79)
  n5 = call "Next Instance Number.vi"("Module Type"="Module Type", "Operation"=Module_Instance_Number_Operation_Enum."Next Instance Number") -> ("Instance Number"=w3:i32)  [unwired: 8 in, 1 out]
  n6 = case "Dropped Module" shown="\"Feed\"" "Module Type" {
    tunnel: "State in" -> [w18 w35 w52 w69 w86 w103 w120 w136 w155 w173 w191 w212 w233 w254 w275]
    tunnel: [w17 w34 w51 w68 w85 w102 w119 w137 w154 w172 w190 w211 w232 w253 w275] -> w2
    tunnel: [w28 w45 w62 w79 w97 w114 w131 w149 w167 w185 w192 w213 w234 w255 T79 {"Module VI Filepath"=path "", "Process Name"="", "Main UI Message Queue"=refnum, "Drop Coords"={"Horizontal"=0, "Vertical"=0}, "Module Parameters"=variant, "Name of Parent Window"=""} ("Drop Parameters")] -> w16
    tunnel: w13 -> [w27 w44 w61 w78 w96 w113 w130 w148 w166 w184 w196 w217 w238 w259 _]
    tunnel: w8 -> [w26 w43 w60 w77 w95 w112 w129 w147 w165 w183 w195 w216 w237 w258 _]
    tunnel: w6 -> [w24 w41 w58 w75 w93 w110 w127 w145 w163 w181 w194 w215 w236 w257 _]
    tunnel: w3 -> [w19 w36 w54 w71 w89 w106 w123 w139 w157 w175 w193 w214 w235 w256 _]
    frame "Feed" {
      w29 = "FD%d"  # Process Name
      n7 = Format Into String(format string=w29, w19) -> (resulting string=w23:string)  [unwired: 2 in, 1 out]
      n8 = Bundle By Name(cluster=T19 {"GUID"="", "Drop Coords"={"Horizontal"=0, "Vertical"=0}, "Process Name"="", "User name"="", "Queue Name"="", "Settings"={"Cycle Period"=500.0, "Ismatech"={"VISA resource name"="", "Simulated?"=TRUE, "Pump Number"=1.0, "Reverse?"=FALSE}, "Masterflex"={"VISA resource name"="", "Simulated?"=TRUE, "Pump Number"=1.0, "Reverse?"=FALSE}, "Mettler"={"VISA resource name"="", "Simulated?"=FALSE}, "Bronkhorst M13 Flow Meter"={"VISA resource name"="", "Simulated?"=TRUE, "Smoothing Steps"=1}, "PID 2 Parameters"={"Input Device"=enum."Default", "Output Device"=enum."Default", "Setpoint"=0.0, "PID gains"={"proportional gain (Kc)"=1.0, "integral time (Ti, min)"=0.01, "derivative time (Td, min)"=0.0}}, "Manual Entry"=0.0, "Auto?"=TRUE, "PID range"={"PID High"=100.0, "PID Low"=0.0, "High Warning"=100.0}, "Tacmina Settings"={"Analog DAQ Task"="", "Digital DAQ Task"=""}, "KNF SIMDOS Settings"={"VISA resource name"="", "Simulated?"=TRUE}, "ASIA Pump C"={"ASIA Pump #"=0, "channel"=0, "Simulated"=FALSE}, "VICI Settings"={"VISA resource name"="", "Pump ID"="", "Pump Head Vol"=0.0, "Reverse?"=FALSE, "Simulated?"=TRUE}, "FLOM Settings"={"VISA resource name"="", "Simulated?"=TRUE, "Pump Number"=0.0}, "SSI PR/LD Settings"={"VISA resource name"="", "Simulated?"=FALSE}, "Masterflex 75211 Settings"={"Analog DAQ Task"="", "Digital DAQ Task"=""}, "SSI P40 Settings"={"VISA resource name"="", "Simulated?"=TRUE}, "Ismatech 3 Channel Settings"={"VISA resource name"="", "Pump Number"=1, "Channel Number"=0, "Simulated?"=TRUE, "Reverse?"=FALSE}, "Bronkhorst M14 Settings"={"VISA resource name"="", "Simulated?"=FALSE, "Smoothing Steps"=1}, "Reset Totalizer"=FALSE, "Input Num Alarm Settings"=[], "Control Type"=enum."g/min", "Front End Display Options"={"Temperature"=TRUE, "Scale Grams"=FALSE, "Density"=TRUE, "Flow (g/min)"=FALSE, "Flow (ml/min)"=TRUE, "PSIG"=TRUE, "Total Grams"=TRUE, "Updated"=TRUE}}, "Settings Load Count"=0, "OP Load Count"=0} ("Feed Module Config"), "GUID"=w27, "Drop Coords"=w24, "Process Name"=w23) -> (w22:T19)
      n9 = in-place {
        in-place-border: w22 -> [w33]
        n10 = in-place-cluster #1(w18) -> ("Main Config.Feed Module Configs"=w32:T19[])
        n11 = Build Array (concatenate)(w32, w33) -> (w31:T19[])
        n12 = in-place-cluster #1("Main Config.Feed Module Configs"=w31) -> (w17:T2)
      }
      n13 = vi-ref "Feed Module (Main).vi"() -> (w21:refnum<vi>)
      n14 = property class="VI Interface Type 0"(reference=w21) -> ("Path"=w20:path)  [unwired: 1 in, 2 out]
      n15 = To Variant(anything=w22) -> (Variant=w25:variant)
      n16 = Bundle By Name(cluster=w26, "Module VI Filepath"=w20, "Module Parameters"=w25, "Process Name"=w23) -> (w28:T79)
    }
    frame "PR" {
      w46 = "PR%d"  # Process Name
      n17 = Format Into String(format string=w46, w36) -> (resulting string=w40:string)  [unwired: 2 in, 1 out]
      n18 = Bundle By Name(cluster=T65 {"GUID"="", "Drop Coords"={"Horizontal"=0, "Vertical"=0}, "Process Name"="", "User name"="", "Queue Name"="", "Settings"={"Cycle Period"=500.0, "PID 2 Parameters"={"Input Device"=enum."Default", "Output Device"=enum."Default", "Setpoint"=0.0, "PID gains"={"proportional gain (Kc)"=1.0, "integral time (Ti, min)"=0.01, "derivative time (Td, min)"=0.0}, "output range"={"output low"=0.0, "output high"=100.0}}, "Manual Entry"=0.0, "Auto?"=TRUE, "4-20mA Input Settings"={"Input Channel "=0}, "4-20mA Out Settings"={"Output DAQ Task"=""}, "Input Channel Tag Name "=""}, "Settings Load Count"=0} ("PRM Config"), "GUID"=w44, "Drop Coords"=w41, "Process Name"=w40) -> (w39:T65)
      n19 = in-place {
        in-place-border: w39 -> [w50]
        n20 = in-place-cluster #2(w35) -> ("Main Config.PR Module Configs"=w49:T65[])
        n21 = Build Array (concatenate)(w49, w50) -> (w48:T65[])
        n22 = in-place-cluster #2("Main Config.PR Module Configs"=w48) -> (w34:T2)
      }
      n23 = vi-ref "4-20mA Module (Main).vi"() -> (w38:refnum<vi>)
      n24 = property class="VI Interface Type 0"(reference=w38) -> ("Path"=w37:path)  [unwired: 1 in, 2 out]
      n25 = To Variant(anything=w39) -> (Variant=w42:variant)
      n26 = Bundle By Name(cluster=w43, "Module VI Filepath"=w37, "Module Parameters"=w42, "Process Name"=w40) -> (w45:T79)
    }
    frame "Scale" {
      w63 = "SM%d"  # Process Name
      n27 = Format Into String(format string=w63, w54) -> (resulting string=w57:string)  [unwired: 2 in, 1 out]
      n28 = Bundle By Name(cluster=T43 {"GUID"="", "Drop Coords"={"Horizontal"=0, "Vertical"=0}, "Process Name"="", "User name"="", "Queue Name"="", "Settings"={"Cycle Period"=500.0, "Mettler"={"VISA resource name"="", "Simulated?"=TRUE}, "Scale Type"=""}, "Load Count"=0} ("Scale Module Config"), "GUID"=w61, "Drop Coords"=w58, "Process Name"=w57) -> (w53:T43)
      n29 = in-place {
        in-place-border: w53 -> [w67]
        n30 = in-place-cluster #3(w52) -> ("Main Config.Scale Module Configs"=w66:T43[])
        n31 = Build Array (concatenate)(w66, w67) -> (w65:T43[])
        n32 = in-place-cluster #3("Main Config.Scale Module Configs"=w65) -> (w51:T2)
      }
      n33 = vi-ref "Scale Module (Main).vi"() -> (w56:refnum<vi>)
      n34 = property class="VI Interface Type 0"(reference=w56) -> ("Path"=w55:path)  [unwired: 1 in, 2 out]
      n35 = To Variant(anything=w53) -> (Variant=w59:variant)
      n36 = Bundle By Name(cluster=w60, "Module VI Filepath"=w55, "Module Parameters"=w59, "Process Name"=w57) -> (w62:T79)
    }
    frame "Flow" {
      w80 = "FL%d"  # Process Name
      n37 = Format Into String(format string=w80, w71) -> (resulting string=w74:string)  [unwired: 2 in, 1 out]
      n38 = Bundle By Name(cluster=T49 {"GUID"="", "Drop Coords"={"Horizontal"=0, "Vertical"=0}, "Process Name"="", "User name"="", "Queue Name"="", "Settings"={"Cycle Period"=500.0, "Flow Meter Type"="", "Bronkhorst M13 Settings"={"VISA resource name"="", "Simulated?"=TRUE, "Smoothing Steps"=1}, "Bronkhorst M14 Settings"={"VISA resource name"="", "Simulated?"=FALSE, "Smoothing Steps"=1}, "Reset Totalizer"=FALSE}, "Load Count"=0} ("Scale Module Config"), "GUID"=w78, "Drop Coords"=w75, "Process Name"=w74) -> (w70:T49)
      n39 = in-place {
        in-place-border: w70 -> [w84]
        n40 = in-place-cluster #4(w69) -> ("Main Config.Flow Module Configs"=w83:T49[])
        n41 = Build Array (concatenate)(w83, w84) -> (w82:T49[])
        n42 = in-place-cluster #4("Main Config.Flow Module Configs"=w82) -> (w68:T2)
      }
      n43 = vi-ref "Flow Module.lvlib:Flow Module (Main).vi"() -> (w73:refnum<vi>)
      n44 = property class="VI Interface Type 0"(reference=w73) -> ("Path"=w72:path)  [unwired: 1 in, 2 out]
      n45 = To Variant(anything=w70) -> (Variant=w76:variant)
      n46 = Bundle By Name(cluster=w77, "Module VI Filepath"=w72, "Module Parameters"=w76, "Process Name"=w74) -> (w79:T79)
    }
    frame "Pump" {
      w87 = T45 {"GUID"="", "Drop Coords"={"Horizontal"=0, "Vertical"=0}, "Process Name"="", "User name"="", "Queue Name"="", "Settings"={"Cycle Period"=500.0, "Manual Entry"=0.0, "Output Device"=enum."Default", "Ismatech"={"VISA resource name"="", "Simulated?"=TRUE, "Pump Number"=1.0, "Reverse?"=FALSE}, "Ismatech 3 Channel Settings"={"VISA resource name"="", "Pump Number"=1, "Channel Number"=0, "Simulated?"=TRUE, "Reverse?"=FALSE}, "Masterflex"={"VISA resource name"="", "Simulated?"=TRUE, "Pump Number"=1.0, "Reverse?"=FALSE}, "VICI Settings"={"VISA resource name"="", "Pump ID"="", "Pump Head Vol"=0.0, "Reverse?"=FALSE, "Simulated?"=TRUE}, "Tacmina Settings"={"Analog DAQ Task"="", "Digital DAQ Task"=""}, "KNF SIMDOS Settings"={"VISA resource name"="", "Simulated?"=TRUE}, "ASIA Pump C"={"ASIA Pump #"=0, "channel"=0, "Simulated"=FALSE}, "FLOM Settings"={"VISA resource name"="", "Simulated?"=TRUE, "Pump Number"=0.0}, "SSI PR/LD Settings"={"VISA resource name"="", "Simulated?"=FALSE}, "SSI P40 Settings"={"VISA resource name"="", "Simulated?"=FALSE}, "Masterflex 75211 Settings"={"Analog DAQ Task"="", "Digital DAQ Task"=""}, "Pump Calibration File"=path "", "Calibration Slope"=0.0, "Calibration Y Intercept"=0.0, "Pump Cal Enum"=0, "Reset Totalizer"=FALSE}, "Load Count"=0}  # Pump Module Config
      w98 = "PM%d"  # Process Name
      n47 = Format Into String(format string=w98, w89) -> (resulting string=w92:string)  [unwired: 2 in, 1 out]
      n48 = Bundle By Name(cluster=w87, "GUID"=w96, "Drop Coords"=w93, "Process Name"=w92) -> (w88:T45)
      n49 = in-place {
        in-place-border: w88 -> [w101]
        n50 = in-place-cluster #5(w86) -> ("Main Config.Pump Module Configs"=w100:T45[])
        n51 = Build Array (concatenate)(w100, w101) -> (w99:T45[])
        n52 = in-place-cluster #5("Main Config.Pump Module Configs"=w99) -> (w85:T2)
      }
      n53 = vi-ref "Pump Module (Main).vi"() -> (w91:refnum<vi>)
      n54 = property class="VI Interface Type 0"(reference=w91) -> ("Path"=w90:path)  [unwired: 1 in, 2 out]
      n55 = To Variant(anything=w88) -> (Variant=w94:variant)
      n56 = Bundle By Name(cluster=w95, "Module VI Filepath"=w90, "Module Parameters"=w94, "Process Name"=w92) -> (w97:T79)
    }
    frame "DO" {
      w104 = T60 {"GUID"="", "Drop Coords"={"Horizontal"=0, "Vertical"=0}, "Process Name"="", "User name"="", "Queue Name"="", "Settings"={"Valve Settings"={"D-O Settings"={"DAQmx Task Name"="", "Output Channel"=0, "Output Channel Names"=[]}, "VICI Electronic Actuator"={"VISA resource name"="", "Mode"=enum."Two Positions With Stops", "Simulated"=FALSE}}, "Valve Type"=enum."Default", "Time On (Sec)"=0.0, "Time Off (Sec)"=0.0, "Run?"=FALSE}, "Load Count"=0}  # D-O Module Config
      w115 = "DO%d"  # Process Name
      # "DO Module (Main).vit"
      n57 = Format Into String(format string=w115, w106) -> (resulting string=w109:string)  [unwired: 2 in, 1 out]
      n58 = Bundle By Name(cluster=w104, "GUID"=w113, "Drop Coords"=w110, "Process Name"=w109) -> (w105:T60)
      n59 = in-place {
        in-place-border: w105 -> [w118]
        n60 = in-place-cluster #6(w103) -> ("Main Config.DO Module Configs"=w116:T60[])
        n61 = Build Array (concatenate)(w116, w118) -> (w117:T60[])
        n62 = in-place-cluster #6("Main Config.DO Module Configs"=w117) -> (w102:T2)
      }
      n63 = vi-ref "D-O Module.lvlib:D-O Module (Main).vi"() -> (w108:refnum<vi>)
      n64 = property class="VI Interface Type 0"(reference=w108) -> ("Path"=w107:path)  [unwired: 1 in, 2 out]
      n65 = To Variant(anything=w105) -> (Variant=w111:variant)
      n66 = Bundle By Name(cluster=w112, "Module VI Filepath"=w107, "Module Parameters"=w111, "Process Name"=w109) -> (w114:T79)
    }
    frame "TCU" {
      w121 = T51 {"GUID"="", "Drop Coords"={"Horizontal"=0, "Vertical"=0}, "Process Name"="", "User name"="", "Queue Name"="", "Settings"={"Cycle Period"=500.0, "Setpoint Entry"=0.0, "Output Device"=enum."Default", "Huber Ministat 230 Settings"={"VISA resource name"="", "Simulated?"=FALSE}, "Lauda Settings"={"VISA resource name"="", "Simulated?"=FALSE, "Pump Power"=2}, "Julabo FP-50 Settings"={"VISA resource name"="", "Simulated?"=FALSE, "Pump Power"=2}, "Internal Control?"=FALSE, "Huber Unistat 410 Settings"={"VISA resource name"="", "Address"=0, "Simulated?"=FALSE}}, "Load Count"=0, "Power Level Changed"=FALSE}  # TCU Module Config
      w132 = "TC%d"  # Process Name
      # "Pump Module (Main).vit"
      n67 = Format Into String(format string=w132, w123) -> (resulting string=w126:string)  [unwired: 2 in, 1 out]
      n68 = Bundle By Name(cluster=w121, "GUID"=w130, "Drop Coords"=w127, "Process Name"=w126) -> (w122:T51)
      n69 = in-place {
        in-place-border: w122 -> [w135]
        n70 = in-place-cluster #7(w120) -> ("Main Config.TCU Module Configs"=w134:T51[])
        n71 = Build Array (concatenate)(w134, w135) -> (w133:T51[])
        n72 = in-place-cluster #7("Main Config.TCU Module Configs"=w133) -> (w119:T2)
      }
      n73 = vi-ref "TCU Module.lvlib:TCU Module (Main).vi"() -> (w125:refnum<vi>)
      n74 = property class="VI Interface Type 0"(reference=w125) -> ("Path"=w124:path)  [unwired: 1 in, 2 out]
      n75 = To Variant(anything=w122) -> (Variant=w128:variant)
      n76 = Bundle By Name(cluster=w129, "Module VI Filepath"=w124, "Module Parameters"=w128, "Process Name"=w126) -> (w131:T79)
    }
    frame "TT" {
      w150 = "TT%d"  # Prefix
      # "TT (Main).vit"
      n77 = Format Into String(format string=w150, w139) -> (resulting string=w144:string)  [unwired: 2 in, 1 out]
      n78 = call "Default Numeric Alarms (TT).vi"() -> ("Default Numeric Alarms"=w138:T38[])  [unwired: 11 in]
      n79 = Bundle By Name(cluster=T39 {"GUID"="", "Drop Coords"={"Horizontal"=0, "Vertical"=0}, "Input Channel Tag Name "="", "Process Name"="", "User name"="", "Queue Name"="", "Input Channel Numeric Alarm Settings"=[]} ("TT Module Config"), "GUID"=w148, "Drop Coords"=w145, "Process Name"=w144, "Input Channel Numeric Alarm Settings"=w138) -> (w142:T39)
      n80 = in-place {
        in-place-border: w142 -> [w153]
        n81 = in-place-cluster #8(w136) -> ("Main Config.TT Module Configs"=w152:T39[])
        n82 = Build Array (concatenate)(w152, w153) -> (w151:T39[])
        n83 = in-place-cluster #8("Main Config.TT Module Configs"=w151) -> (w137:T2)
      }
      n84 = vi-ref "TT (Main).vi"() -> (w141:refnum<vi>)
      n85 = property class="VI Interface Type 0"(reference=w141) -> ("Path"=w140:path)  [unwired: 1 in, 2 out]
      n86 = To Variant(anything=w142) -> (Variant=w146:variant)
      n87 = Bundle By Name(cluster=w147, "Module VI Filepath"=w140, "Module Parameters"=w146, "Process Name"=w144) -> (w149:T79)
    }
    frame "U3" {
      w168 = "U3%d"  # Prefix
      # "U3 (Main).vit"
      n88 = Format Into String(format string=w168, w157) -> (resulting string=w162:string)  [unwired: 2 in, 1 out]
      n89 = call "Default Numeric Alarms (TT).vi"() -> ("Default Numeric Alarms"=w156:T38[])  [unwired: 11 in]
      n90 = Bundle By Name(cluster=T47 {"GUID"="", "Drop Coords"={"Horizontal"=0, "Vertical"=0}, "AI Channel Number"=enum."Default", "Process Name"="", "User name"="", "Queue Name"="", "Input Channel Numeric Alarm Settings"=[]} ("TT Module Config"), "GUID"=w166, "Drop Coords"=w163, "Process Name"=w162, "Input Channel Numeric Alarm Settings"=w156) -> (w160:T47)
      n91 = in-place {
        in-place-border: w160 -> [w171]
        n92 = in-place-cluster #9(w155) -> ("Main Config.U3 Module Configs"=w170:T47[])
        n93 = Build Array (concatenate)(w170, w171) -> (w169:T47[])
        n94 = in-place-cluster #9("Main Config.U3 Module Configs"=w169) -> (w154:T2)
      }
      n95 = vi-ref "U3 Module.lvlib:U3 (Main).vit"() -> (w159:refnum<vi>)
      n96 = property class="VI Interface Type 3"(reference=w159) -> ("Path"=w158:path)  [unwired: 1 in, 2 out]
      n97 = To Variant(anything=w160) -> (Variant=w164:variant)
      n98 = Bundle By Name(cluster=w165, "Module VI Filepath"=w158, "Module Parameters"=w164, "Process Name"=w162) -> (w167:T79)
    }
    frame "PT" {
      w186 = "PT%d"  # Process Name
      n99 = Format Into String(format string=w186, w175) -> (resulting string=w180:string)  [unwired: 2 in, 1 out]
      n100 = call "Default Numeric Alarms (TT).vi"() -> ("Default Numeric Alarms"=w174:T38[])  [unwired: 11 in]
      n101 = Bundle By Name(cluster=T42 {"GUID"="", "Drop Coords"={"Horizontal"=0, "Vertical"=0}, "Input Channel Tag Name "="", "Process Name"="", "User name"="", "Queue Name"="", "Input Channel Numeric Alarm Settings"=[]} ("TT Module Config"), "GUID"=w184, "Drop Coords"=w181, "Process Name"=w180, "Input Channel Numeric Alarm Settings"=w174) -> (w178:T42)
      n102 = in-place {
        in-place-border: w178 -> [w189]
        n103 = in-place-cluster #10(w173) -> ("Main Config.PT Module Configs"=w188:T42[])
        n104 = Build Array (concatenate)(w188, w189) -> (w187:T42[])
        n105 = in-place-cluster #10("Main Config.PT Module Configs"=w187) -> (w172:T2)
      }
      n106 = vi-ref "PT (Main).vi"() -> (w177:refnum<vi>)
      n107 = property class="VI Interface Type 0"(reference=w177) -> ("Path"=w176:path)  [unwired: 1 in, 2 out]
      n108 = To Variant(anything=w178) -> (Variant=w182:variant)
      n109 = Bundle By Name(cluster=w183, "Module VI Filepath"=w176, "Module Parameters"=w182, "Process Name"=w180) -> (w185:T79)
    }
    frame "OPC" {
      n110 = in-place {
        in-place-border: w196 -> [w209]
        in-place-border: w195 -> [w208]
        in-place-border: w194 -> [w206]
        in-place-border: w193 -> [w202]
        in-place-border: [w199] -> w192
        w210 = "OP%d"  # Process Name
        n111 = in-place-cluster #11(w191) -> ("Main Config.OPC Module Configs"=w198:T9[])
        n112 = Format Into String(format string=w210, w202) -> (resulting string=w205:string)  [unwired: 2 in, 1 out]
        n113 = Bundle By Name(cluster=T9 {"State"=enum."Idle", "GUID"="", "Process Name"="", "User name"="", "Drop Coords"={"Horizontal"=0, "Vertical"=0}, "Configuration"={"Cycle Period"=500.0, "server endpoint URL"="", "security policy"={"message mode"=enum."None", "security"=enum."Basic256"}, "Trust Any Server"=TRUE}, "First Iteration"=FALSE, "Data"=[], "Load Count"=0, "Log Started"=FALSE, "subscription ID out"=0, "OPC UA client refnum out"="", "Event Registration Refnum"=refnum, "Start Time"=timestamp(0 s since 1904-01-01), "Current Time"=timestamp(0 s since 1904-01-01), "Tag Data"=[]} ("OPC Module Config"), "GUID"=w209, "Drop Coords"=w206, "Process Name"=w205) -> (w204:T9)
        n114 = vi-ref "OPC Main.vi"() -> (w201:refnum<vi>)
        n115 = property class="VI Interface Type 0"(reference=w201) -> ("Path"=w203:path)  [unwired: 1 in, 2 out]
        n116 = To Variant(anything=w204) -> (Variant=w207:variant)
        n117 = Build Array (concatenate)(w198, w204) -> (w197:T9[])
        n118 = in-place-cluster #11("Main Config.OPC Module Configs"=w197) -> (w190:T2)
        n119 = Bundle By Name(cluster=w208, "Module VI Filepath"=w203, "Module Parameters"=w207, "Process Name"=w205) -> (w199:T79)
      }
    }
    frame "SC" {
      n120 = in-place {
        in-place-border: w217 -> [w230]
        in-place-border: w216 -> [w229]
        in-place-border: w215 -> [w227]
        in-place-border: w214 -> [w223]
        in-place-border: [w221] -> w213
        w231 = "SC%d"  # Process Name
        n121 = in-place-cluster #12(w212) -> ("Main Config.SC Module Configs"=w220:T69[])
        n122 = Format Into String(format string=w231, w223) -> (resulting string=w226:string)  [unwired: 2 in, 1 out]
        n123 = Bundle By Name(cluster=T69 {"GUID"="", "Drop Coords"={"Horizontal"=0, "Vertical"=0}, "Process Name"="", "User name"="", "Queue Name"="", "Settings"={"Cycle Period"=500.0, "Sonicator Type"="", "SS P100 Settings"={"VISA resource name"="", "Simulated?"=FALSE}, "Setpoint (µm)"=0.0, "Cutoff (W)"=0.0}, "Load Count"=0} ("Sonicator Module Config"), "GUID"=w230, "Drop Coords"=w227, "Process Name"=w226) -> (w225:T69)
        n124 = vi-ref "Sonicator Module.lvlib:Sonicator Module (Main).vi"() -> (w222:refnum<vi>)
        n125 = property class="VI Interface Type 0"(reference=w222) -> ("Path"=w224:path)  [unwired: 1 in, 2 out]
        n126 = To Variant(anything=w225) -> (Variant=w228:variant)
        n127 = Build Array (concatenate)(w220, w225) -> (w219:T69[])
        n128 = in-place-cluster #12("Main Config.SC Module Configs"=w219) -> (w211:T2)
        n129 = Bundle By Name(cluster=w229, "Module VI Filepath"=w224, "Module Parameters"=w228, "Process Name"=w226) -> (w221:T79)
      }
    }
    frame "AM" {
      n130 = in-place {
        in-place-border: w238 -> [w251]
        in-place-border: w237 -> [w250]
        in-place-border: w236 -> [w248]
        in-place-border: w235 -> [w244]
        in-place-border: [w242] -> w234
        w252 = "AM%d"  # Process Name
        n131 = in-place-cluster #13(w233) -> ("Main Config.AM Module Configs"=w241:T72[])
        n132 = Format Into String(format string=w252, w244) -> (resulting string=w247:string)  [unwired: 2 in, 1 out]
        n133 = Bundle By Name(cluster=T72 {"GUID"="", "Drop Coords"={"Horizontal"=0, "Vertical"=0}, "Process Name"="", "User name"="", "Queue Name"="", "Settings"={"Cycle Period"=500.0, "Agitator Type"="", "Setpoint (µm)"=0.0, "IKA EUROSTAR Settings"={"VISA resource name"="", "Simulated?"=FALSE}}, "Load Count"=0} ("Sonicator Module Config"), "GUID"=w251, "Drop Coords"=w248, "Process Name"=w247) -> (w246:T72)
        n134 = vi-ref "Agitator Module.lvlib:Agitator Module (Main).vi"() -> (w243:refnum<vi>)
        n135 = property class="VI Interface Type 0"(reference=w243) -> ("Path"=w245:path)  [unwired: 1 in, 2 out]
        n136 = To Variant(anything=w246) -> (Variant=w249:variant)
        n137 = Build Array (concatenate)(w241, w246) -> (w240:T72[])
        n138 = in-place-cluster #13("Main Config.AM Module Configs"=w240) -> (w232:T2)
        n139 = Bundle By Name(cluster=w250, "Module VI Filepath"=w245, "Module Parameters"=w249, "Process Name"=w247) -> (w242:T79)
      }
    }
    frame "CM" {
      n140 = in-place {
        in-place-border: w259 -> [w272]
        in-place-border: w258 -> [w271]
        in-place-border: w257 -> [w269]
        in-place-border: w256 -> [w265]
        in-place-border: [w263] -> w255
        w273 = "CM%d"  # Process Name
        n141 = in-place-cluster #14(w254) -> ("Main Config.CM Module Configs"=w262:T75[])
        n142 = Format Into String(format string=w273, w265) -> (resulting string=w268:string)  [unwired: 2 in, 1 out]
        n143 = Bundle By Name(cluster=T75 {"GUID"="", "Drop Coords"={"Horizontal"=0, "Vertical"=0}, "Process Name"="", "User name"="", "Queue Name"="", "Settings"={"Cycle Period"=500.0, "Manual Entry"=0.0, "Output Device"=enum."Default", "EPOS4 Settings"={"VISA resource name"="", "axis"={"keyHandle"=1, "nodeId"=1}, "Simulated?"=TRUE}}, "Load Count"=0} ("Pump Module Config"), "GUID"=w272, "Drop Coords"=w269, "Process Name"=w268) -> (w267:T75)
        n144 = vi-ref "Centrifuge Module.lvlib:Centrifuge Module (Main).vi"() -> (w264:refnum<vi>)
        n145 = property class="VI Interface Type 0"(reference=w264) -> ("Path"=w266:path)  [unwired: 1 in, 2 out]
        n146 = To Variant(anything=w267) -> (Variant=w270:variant)
        n147 = Build Array (concatenate)(w262, w267) -> (w261:T75[])
        n148 = in-place-cluster #14("Main Config.CM Module Configs"=w261) -> (w253:T2)
        n149 = Bundle By Name(cluster=w271, "Module VI Filepath"=w266, "Module Parameters"=w270, "Process Name"=w268) -> (w263:T79)
      }
    }
    frame Default {
      # "This case should not execute."
    }
  }
  "Drop Parameters" <- w16
  "State out" <- w2
